vi "Format&SaveDataWithAttributes.vi"(0 "Comment":string="This is a test", 1 "Exp_Temperature_K":dbl=5.0, 2 "Det_Mono1_CenterWL_nm":dbl=490.0, 3 "Exc_ExcitationPower_uW":dbl=0.21, 4 "Exc_ExcitationSource":enum16{"P", "CW"}(ring), 5 "Exc_ExcitationWavelength_nm":dbl=450.0, 6 "Det_AcqTime_ms":dbl=500.0, 7 "Det_Mono1_EntSlit_mm":dbl=0.01, 8 "Measurement type":T2(ring)=enum."XY Intensity Map", 9 "Det_Mono1_ExtSlit_mm":dbl=0.01, 10 "Data_PLInt_cts":i32[](array[numeric])=[1, 3, 2, 1], 11 "FileName":string="test", 12 "Data_Wavelength_nm":sgl[](array[numeric])=[490.08, 490.12, 490.16, 490.2], 13 "Acq Mode":T1=enum."Spectrum" caption="Acq mode", 14 "Data_Angle_deg":sgl[](array[numeric])=[490.08, 490.12, 490.16, 490.2], 15 "Log File In":string, 16 "Data_FSMPos_V":dbl[][](array[numeric]), 18 "Data_CCD_px":dbl[][](array[numeric])) -> (17 "Log File Out":string, 25 "WrittenDatasetName":string)   [LabVIEW 2019]
uses:
  TypeDefs/AcqMode.ctl
  <vilib>/UPVI/lvhdf5/dataset.llb/LVH5D Operation.ctl
  <vilib>/Utility/miscctls.llb/LVRectTypeDef.ctl
  <vilib>/UPVI/lvhdf5/attribute.llb/LVH5A Operation.ctl
  <vilib>/UPVI/lvhdf5/group.llb/H5G_obj_t.ctl
  <vilib>/UPVI/lvhdf5/identifier.llb/Not an HDF5 Refnum Constant.vi
  <vilib>/UPVI/lvhdf5/common.llb/To HDF5 Ref.vi
  <vilib>/UPVI/lvhdf5/group.llb/OpenCreateGroup (String).vi
  <vilib>/Utility/VariantDataType/GetClusterInfo.vi
  <vilib>/Utility/VariantDataType/GetTypeInfo.vi
  <vilib>/UPVI/lvhdf5/utility.llb/Select HDF5 Dialog.vi
  <vilib>/UPVI/lvhdf5/utility.llb/Select HDF5 Dialog (Object Only).vi
  <vilib>/UPVI/lvhdf5/dataset.llb/Simple H5Dwrite (Variant).vi
  <vilib>/UPVI/lvhdf5/attribute.llb/Write Multiple Attributes.vi
  <vilib>/UPVI/lvhdf5/dataset.llb/H5Dclose.vi
  <vilib>/UPVI/lvhdf5/dataset.llb/Write Dataset with Attributes.xnode
  <vilib>/UPVI/lvhdf5/library.llb/HDF5 Ref.ctl
  <vilib>/UPVI/lvhdf5/attribute.llb/Cluster to Attribute Array.xnode
  <vilib>/Utility/error.llb/Error Cluster From Error Code.vi
  <vilib>/UPVI/lvhdf5/dataset.llb/OpenCreateReplace Dataset by Element Type.vi
  <vilib>/UPVI/lvhdf5/dataspace.llb/H5Sselect_hyperslab.vi
  <vilib>/UPVI/lvhdf5/dataset.llb/H5Dwrite (Variant).vi
  <vilib>/UPVI/lvhdf5/dataset.llb/H5Dget_space.vi
  <vilib>/UPVI/lvhdf5/attribute.llb/private/LVH5AwriteWDTAttrs.vi
  <vilib>/UPVI/lvhdf5/dataspace.llb/H5Sclose.vi
  <vilib>/UPVI/lvhdf5/file.llb/LVH5F Operation.ctl
  <vilib>/UPVI/lvhdf5/utility.llb/Select HDF5 Dialog (File and Object).vi
  <vilib>/Utility/VariantDataType/VariantType.lvlib
panel:
  in  "Main 3D Data to write":dbl[][][](array[numeric])=[[[2.2, 4.4, 3.3, 5.5, 6.6]]]
  out "File path":path=path "Cluster Attributes.hdf5"
  in  "DatasetName":string="test"
  in  "Main 2D Data to write":dbl[][](array[numeric])=[[2.2, 4.4, 3.3, 5.5, 6.6]]
  out "Date":string="2006-1-11"
  in  "Pol_L/2Exc_deg":dbl[](array[numeric])
  in  "Pol_L/2Det_deg":dbl[](array[numeric])
  in  "MeasurementName":string
  out "Exists":bool
  out "Homonyms":string[](array[string])
  out "size(s)":i32
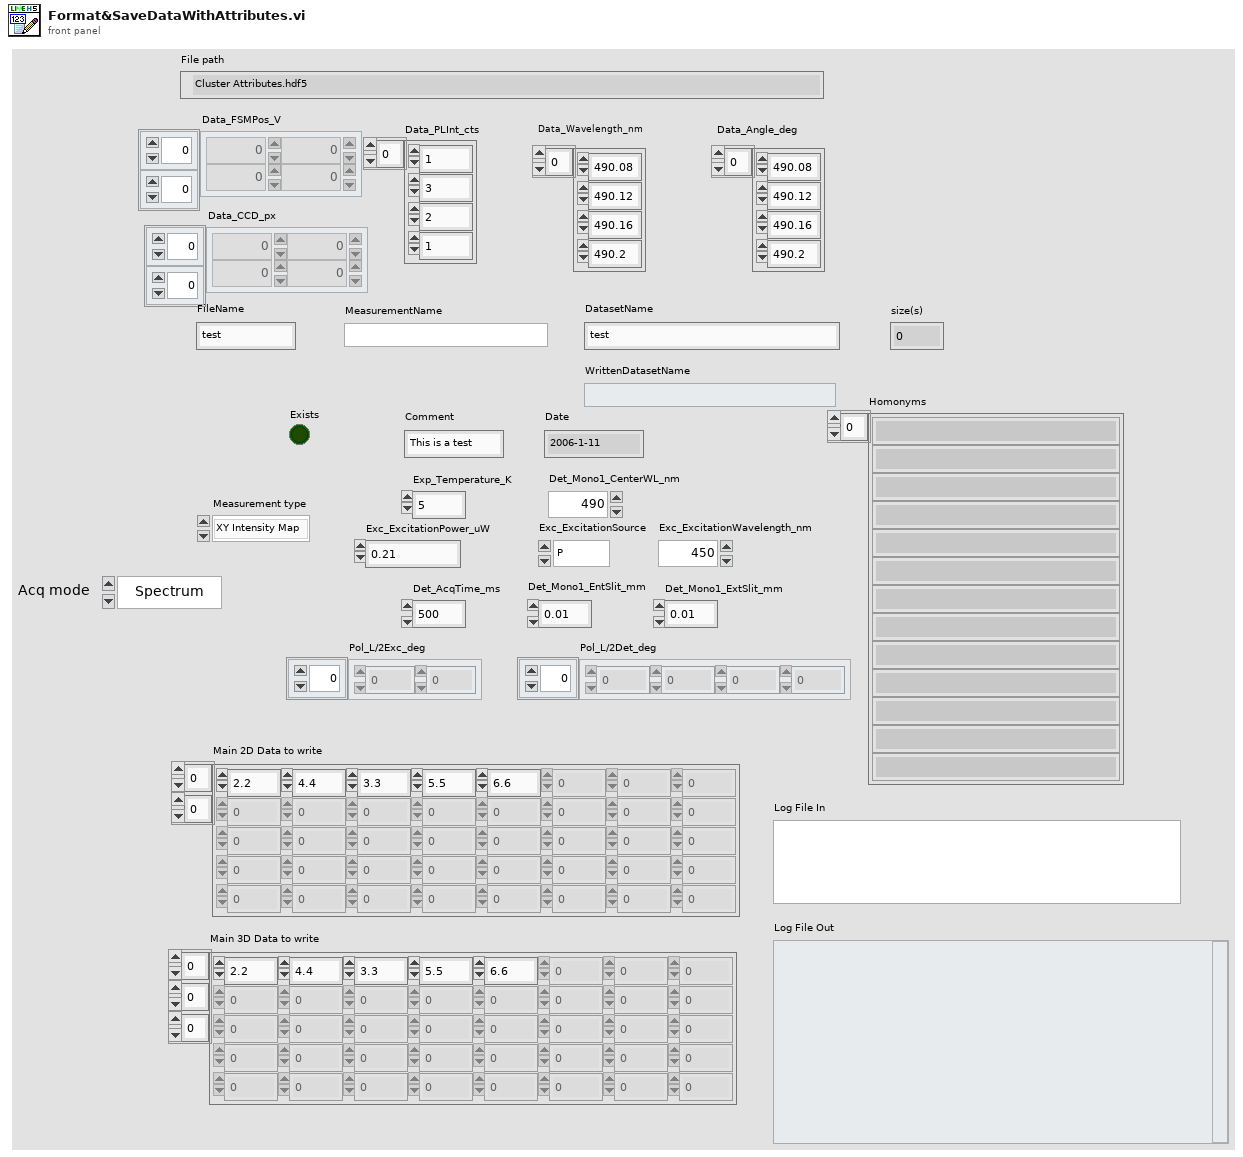
[diagram p1: front panel]
types:
  T1 = typedef "AcqMode.ctl" = enum16{"Image", "Spectrum", "APD 1", "APD 2", "APD 1+2"}
  T2 = enum16{"Contrast", "XY Intensity Map", "Polarisation", "Spectrum"}
  T3 = typedef "LVH5D Operation.ctl" = enum16{"open", "replace", "create", "open or create", "create or replace", "create or replace with confirmation"}
  T4 = typedef "HDF5 Ref.ctl" = refnum<k1>
  T5 = typedef "LVH5A Operation.ctl" = enum16{"open", "replace", "create", "open or create", "create or replace", "create or replace with confirmation"}
  T6 = typedef "LVRectTypeDef.ctl" = cluster{"Left":i16, "Top":i16, "Right":i16, "Bottom":i16}
  T7 = cluster{"Behavior":enum32{"Invalid", "Default", "Floating", "Floating/Auto-Hide", "Modal"}, "Position":T6, "Center":bool, "Title":string}
  T8 = typedef "LVH5F Operation.ctl" = enum16{"open", "open or create", "create or replace", "create or replace (with confirmation)", "create", "open (read only)"}
  T9 = typedef "H5G_obj_t.ctl" = i32
  T10 = cluster{"Object Types (any)":T9[], "Object Pattern":string}
  T11 = cluster{"date/time string":string, "Comment":string, "Exp_Temperature_K":dbl, "Exc_ExcitationSource":enum16{"P", "CW"}, "Exc_ExcitationWavelength_nm":dbl, "Exc_ExcitationPower_uW":dbl, "Det_AcqTime_ms":dbl, "Det_Mono1_EntSlit_mm":dbl, "Det_Mono1_ExtSlit_mm":dbl, "Pol_L/2Exc_deg":dbl[], "Pol_L/2Det_deg":dbl[], "Data_CCD_px":dbl[][]}
  T12 = cluster{"date/time string":string, "Comment":string, "Exp_Temperature_K":dbl, "Exc_ExcitationSource":enum16{"P", "CW"}, "Exc_ExcitationWavelength_nm":dbl, "Exc_ExcitationPower_uW":dbl, "Det_AcqTime_ms":dbl, "Det_Mono1_EntSlit_mm":dbl, "Det_Mono1_ExtSlit_mm":dbl, "Pol_L/2Exc_deg":dbl[], "Pol_L/2Det_deg":dbl[], "Data_Wavelength_nm":sgl[]}
  T13 = cluster{"date/time string":string, "Comment":string, "Exp_Temperature_K":dbl, "Exc_ExcitationSource":enum16{"P", "CW"}, "Exc_ExcitationWavelength_nm":dbl, "Exc_ExcitationPower_uW":dbl, "Det_AcqTime_ms":dbl, "Det_Mono1_EntSlit_mm":dbl, "Det_Mono1_ExtSlit_mm":dbl, "Pol_L/2Exc_deg":dbl[], "Pol_L/2Det_deg":dbl[], "Data_FSMPos_V":dbl[][]}
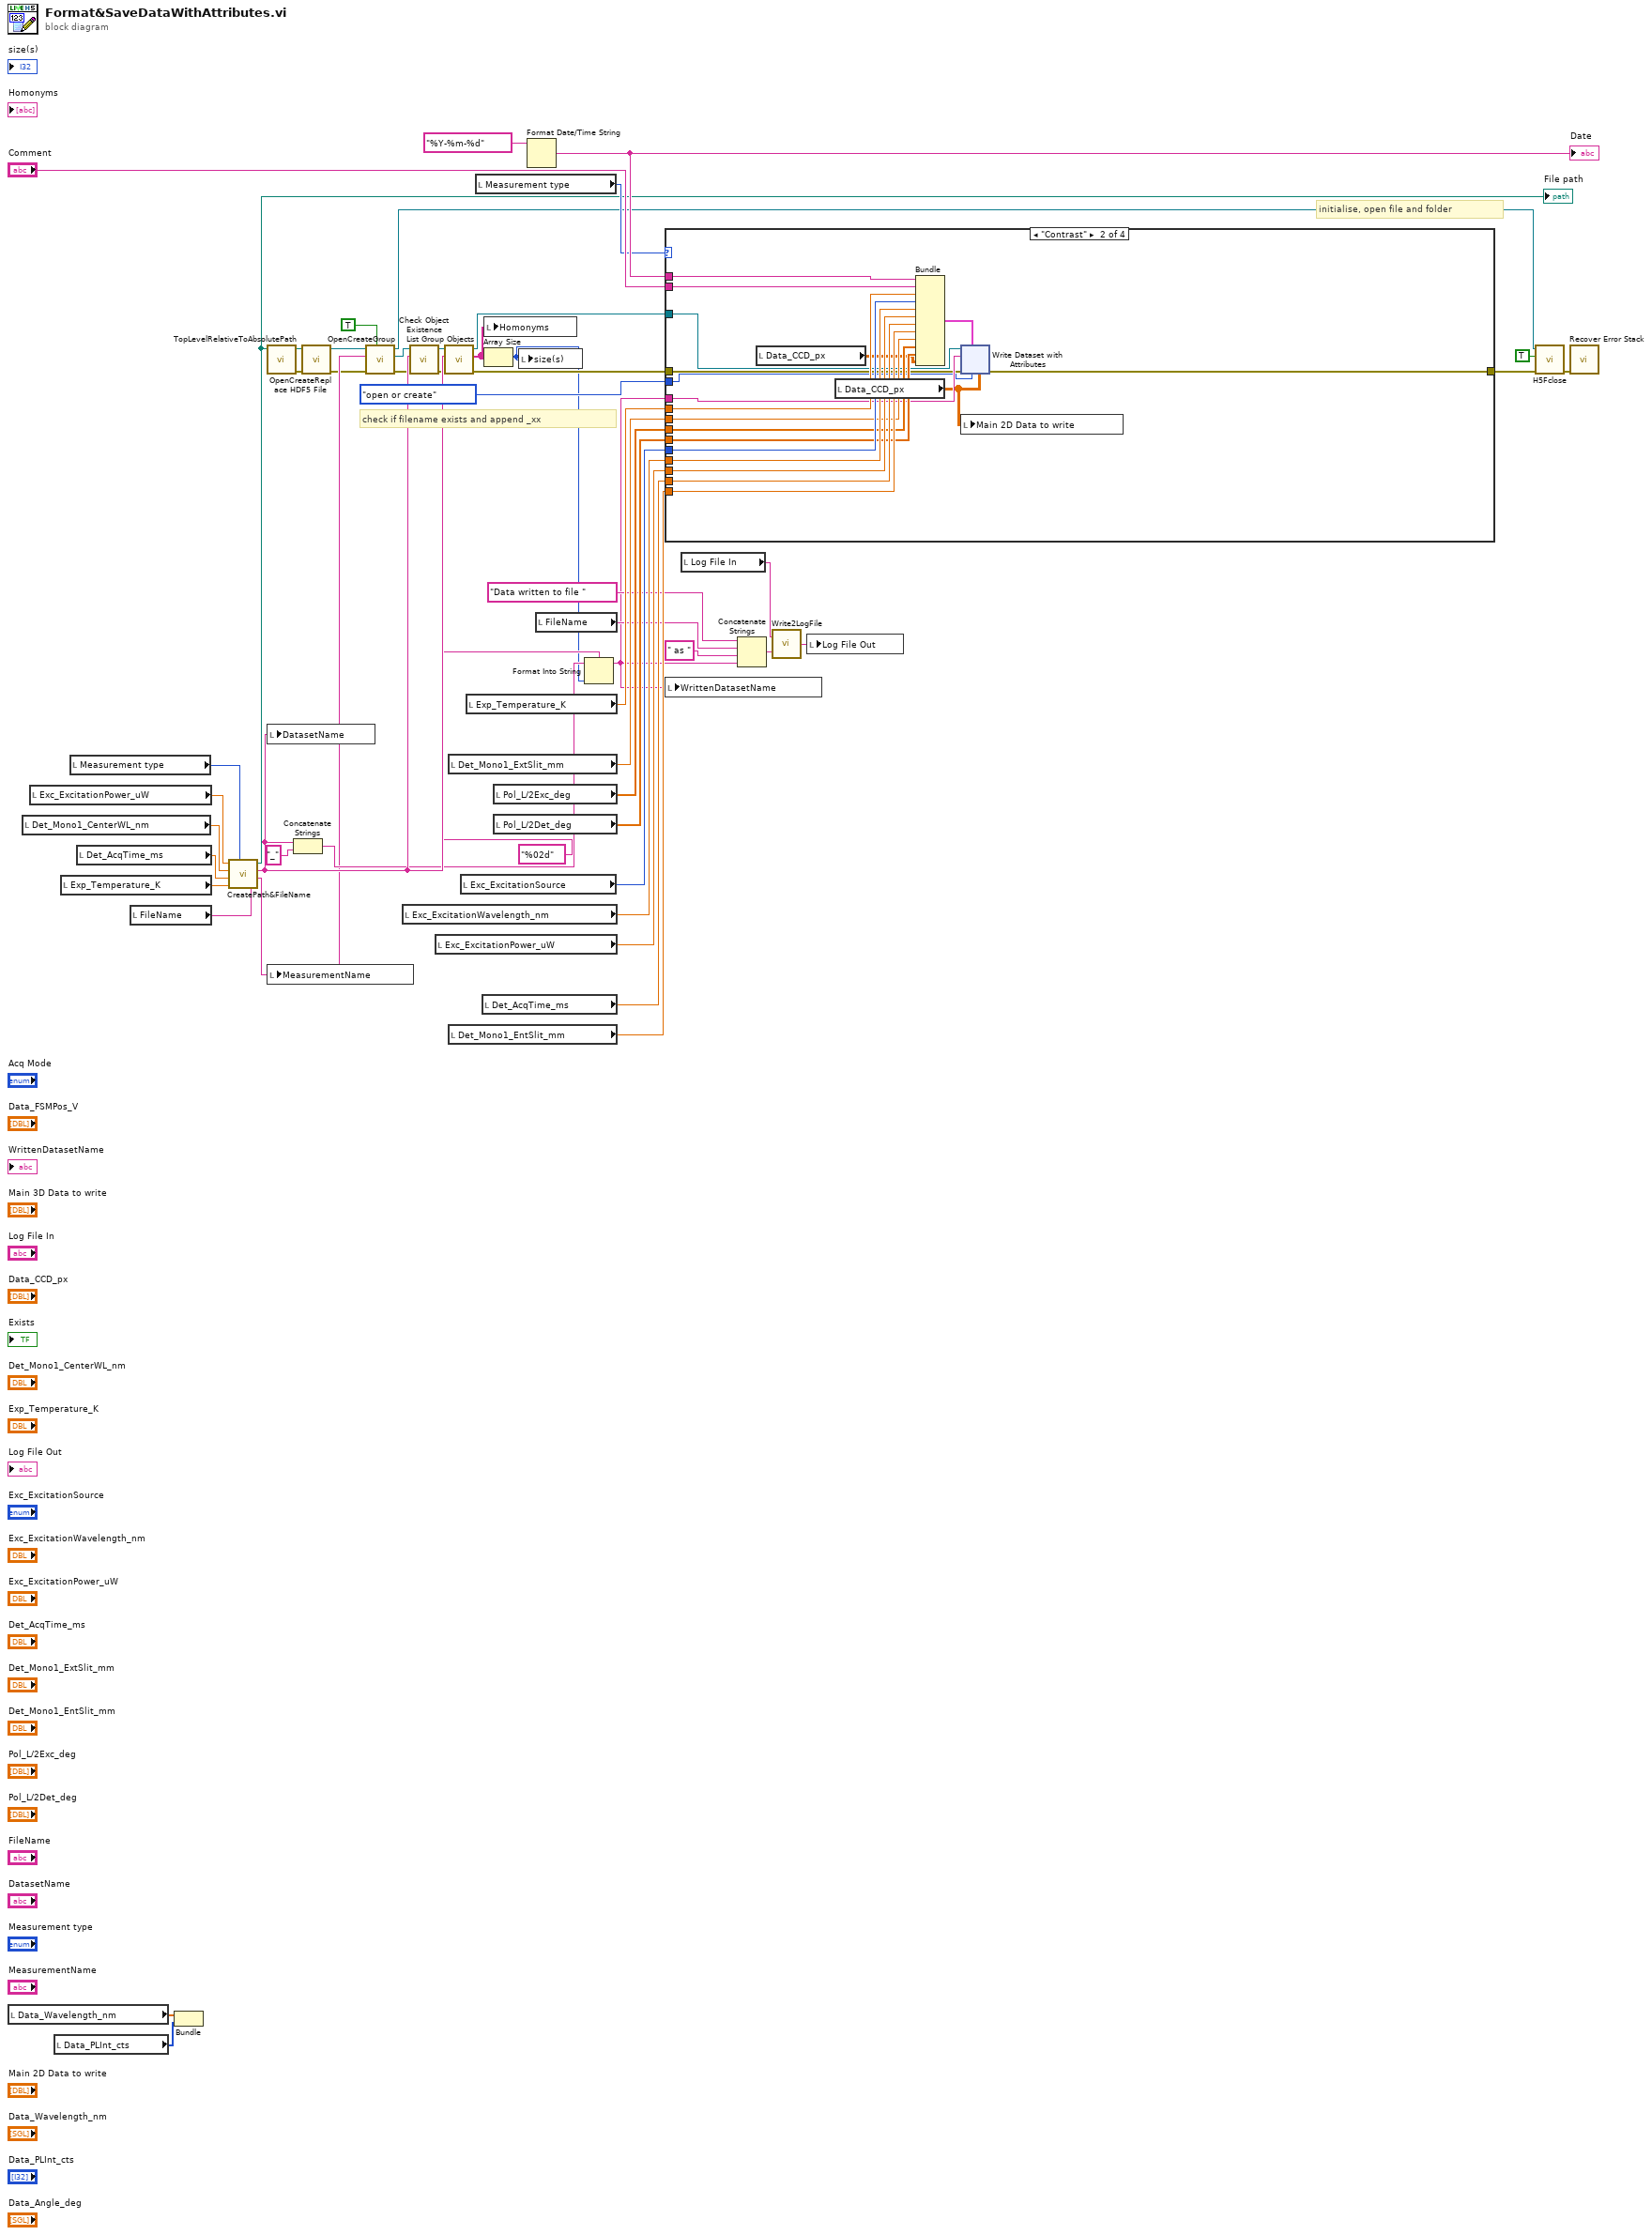
[diagram p0: block diagram]
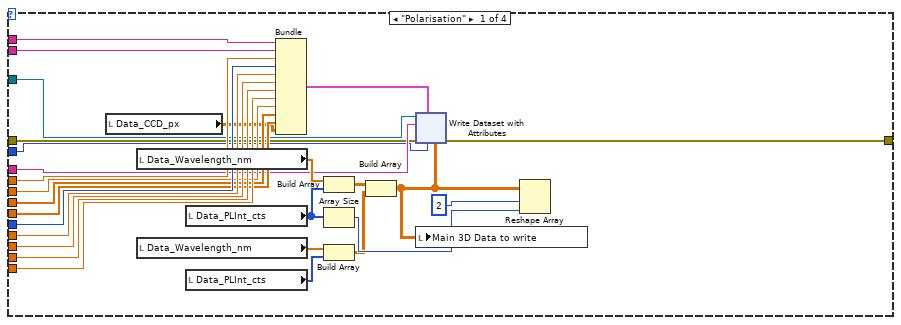
[diagram p2: hidden frame]
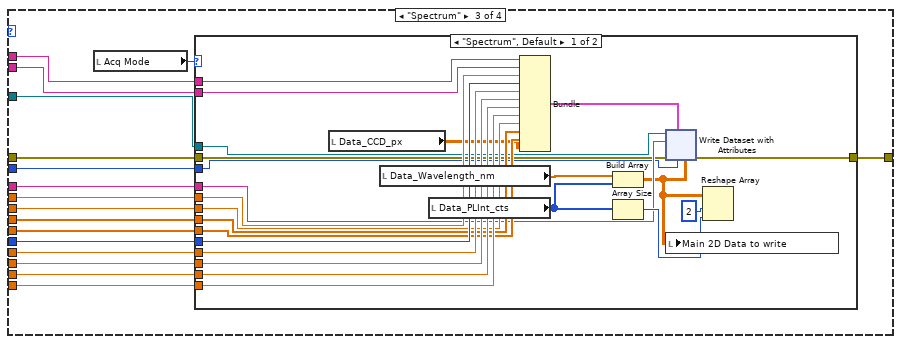
[diagram p3: hidden frame]
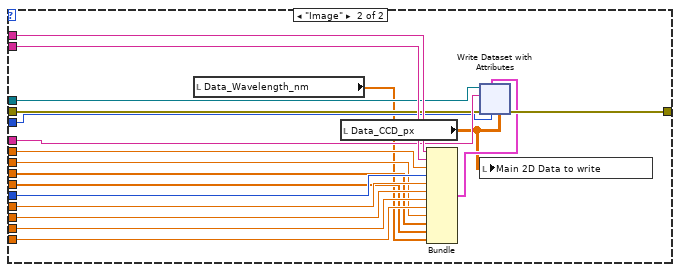
[diagram p4: hidden frame]
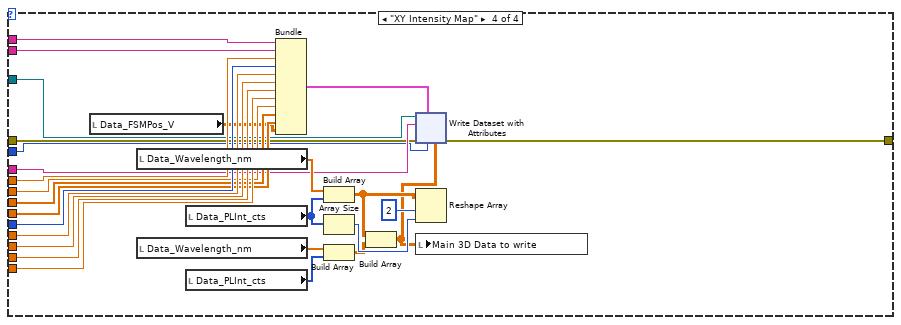
[diagram p5: hidden frame]
diagram:
  # "initialise, open file and folder"
  # "check if filename exists and append _xx"
  n1 = local read "Data_Wavelength_nm"() -> (w12:sgl[])
  n2 = local read "Det_Mono1_CenterWL_nm"() -> (w26:dbl)
  n3 = local read "Exc_ExcitationPower_uW"() -> (w23:dbl)
  n4 = local read "Data_PLInt_cts"() -> (w13:i32[])
  n5 = local read "Exp_Temperature_K"() -> (w24:dbl)
  n6 = local read "Measurement type"() -> (w1:T2)
  n7 = local read "Det_AcqTime_ms"() -> (w22:dbl)
  n8 = local read "FileName"() -> (w21:string)
  n9 = Bundle("Data_Wavelength_nm"=w12, "Data_PLInt_cts"=w13) -> ()  [unwired: 1 in, 1 out]
  n10 = call "CreatePath&FileName.vi"("FileName"=w21, "Measurement type"=w1, "Temp_K"=w24, "AcqTime_ms"=w22, "CenterWL_nm"=w26, "ExcPow_uW"=w23) -> ("MeasurementGroupName"=w25:string, "DatasetName"=w37:string, "File path"=w14:path)
  "File path" <- w14
  n11 = call "TopLevelRelativeToAbsolutePath.vi"("Path Relative to Top Level VI"=w14) -> ("error out"=w10:errorcluster, "Absolute path"=w9:path)  [unwired: 9 in]
  n12 = local write "DatasetName"(w37) -> ()
  n13 = local write "MeasurementName"(w25) -> ()
  n14 = Concatenate Strings(w37, "_" ("string")) -> (w35:string)
  n15 = call <vilib>:"OpenCreateReplace HDF5 File.vi"("error in (no error)"=w10, "path"=w9) -> ("error out"=w16:errorcluster, "HDF5 Ref out"=w15:T4)  [unwired: 6 in]
  n16 = call-poly <vilib>:"OpenCreateGroup.vi"("Create if not found (F)"=TRUE, "error in (no error)"=w16, "Group"=w25, "HDF5 Ref"=w15) -> ("error out"=w29:errorcluster, "HDF5 Group Ref"=w28:T4, "HDF5 Ref out"=w19:T4)  [unwired: 5 in]
  n17 = local read "Exc_ExcitationWavelength_nm"() -> (w42:dbl)
  n18 = call <vilib>:"Check Object Existence.vi"("error in (no error)"=w29, "name"=w37, "HDF5 Ref"=w28) -> ("error out"=w30:errorcluster, "HDF5 Ref out"=w31:T4)  [unwired: 4 in, 1 out]
  n19 = local read "Exc_ExcitationPower_uW"() -> (w43:dbl)
  n20 = call <vilib>:"List Group Objects.vi"("error in (no error)"=w30, "pattern"=w37, "HDF5 Loc Ref"=w31) -> ("error out"=w49:errorcluster, "Object Names"=w32:string[], "HDF5 Loc Ref out"=w51:T4)  [unwired: 3 in, 1 out]
  n21 = local read "Det_Mono1_ExtSlit_mm"() -> (w46:dbl)
  n22 = local read "Det_Mono1_EntSlit_mm"() -> (w45:dbl)
  n23 = local read "Exc_ExcitationSource"() -> (w41:enum16{"P", "CW"})
  n24 = local read "Exp_Temperature_K"() -> (w40:dbl)
  n25 = local read "Measurement type"() -> (w20:T2)
  n26 = local read "Det_AcqTime_ms"() -> (w44:dbl)
  n27 = local write "Homonyms"(w32) -> ()
  n28 = Array Size(array=w32) -> (size(s)=w34:i32)
  n29 = local read "Pol_L/2Exc_deg"() -> (w47:dbl[])
  n30 = local read "Pol_L/2Det_deg"() -> (w48:dbl[])
  n31 = local write "size(s)"(w34) -> ()
  n32 = Format Date/Time String(time format string (%c)="%Y-%m-%d") -> (date/time string=w38:string)  [unwired: 2 in]
  "Date" <- w38
  n33 = local read "FileName"() -> (w7:string)
  n34 = Format Into String(format string="%02d", initial string=w35, w34) -> (resulting string=w5:string)  [unwired: 1 in, 1 out]
  n35 = case shown="\"Contrast\"" w20 {
    tunnel: w38 -> [w75 w414 w747 w1444]
    tunnel: "Comment" -> [w74 w413 w746 w1443]
    tunnel: w40 -> [w73 w412 w745 w1442]
    tunnel: w41 -> [w72 w411 w744 w1441]
    tunnel: w42 -> [w71 w410 w743 w1440]
    tunnel: w43 -> [w70 w409 w742 w1439]
    tunnel: w44 -> [w69 w408 w741 w1438]
    tunnel: w45 -> [w68 w407 w740 w1437]
    tunnel: w46 -> [w67 w406 w739 w1436]
    tunnel: w47 -> [w66 w405 w738 w1435]
    tunnel: w48 -> [w65 w404 w737 w1434]
    tunnel: w5 -> [w64 w403 w736 w1433]
    tunnel: w49 -> [w63 w402 w735 w1432]
    tunnel: LVH5D_Operation."open or create" ("operation (open or create)") -> [w62 w401 w734 w1431]
    tunnel: w51 -> [w61 w400 w733 w1430]
    tunnel: [w60 w399 w732 w1429] -> w52
    frame "Polarisation" {
      n36 = local read "Data_CCD_px"() -> (w59:dbl[][])
      n37 = local read "Data_Wavelength_nm"() -> (w76:sgl[])
      n38 = local read "Data_Wavelength_nm"() -> (w57:sgl[])
      n39 = local read "Data_PLInt_cts"() -> (w77:i32[])
      n40 = local read "Data_PLInt_cts"() -> (w56:i32[])
      n41 = Bundle("date/time string"=w75, "Comment"=w74, "Exp_Temperature_K"=w73, "Exc_ExcitationSource"=w72, "Exc_ExcitationWavelength_nm"=w71, "Exc_ExcitationPower_uW"=w70, "Det_AcqTime_ms"=w69, "Det_Mono1_EntSlit_mm"=w68, "Det_Mono1_ExtSlit_mm"=w67, "Pol_L/2Exc_deg"=w66, "Pol_L/2Det_deg"=w65, "Data_CCD_px"=w59) -> (w58:T11)  [unwired: 1 in]
      n42 = Build Array(w76, w77) -> (w54:sgl[][])
      n43 = Array Size(array=w77) -> (size(s)=w78:i32)
      n44 = Build Array(w57, w56) -> (w55:sgl[][])
      n45 = Build Array(w54, w55) -> (w53:sgl[][][])
      n46 = xnode "Write Dataset with Attributes"("Dataset Path"=w64, "error in (no error)"=w63, "operation (open or create)"=w62, "HDF5 Path or Ref"=w61, "Attribute Value(s)"=w58, "Data"=w53) -> ("error out"=w60:errorcluster)  [unwired: 2 in, 2 out]
      n47 = local write "Main 3D Data to write"(w53) -> ()
      n48 = Reshape Array(w53, 2 ("dimension size"), w78) -> ()  [unwired: 1 out]
    }
    frame "Contrast" {
      n49 = local read "Data_CCD_px"() -> (w398:dbl[][])
      n50 = local read "Data_CCD_px"() -> (w396:dbl[][])
      n51 = Bundle("date/time string"=w414, "Comment"=w413, "Exp_Temperature_K"=w412, "Exc_ExcitationSource"=w411, "Exc_ExcitationWavelength_nm"=w410, "Exc_ExcitationPower_uW"=w409, "Det_AcqTime_ms"=w408, "Det_Mono1_EntSlit_mm"=w407, "Det_Mono1_ExtSlit_mm"=w406, "Pol_L/2Exc_deg"=w405, "Pol_L/2Det_deg"=w404, "Data_CCD_px"=w398) -> (w397:T11)  [unwired: 1 in]
      n52 = xnode "Write Dataset with Attributes"("Dataset Path"=w403, "error in (no error)"=w402, "operation (open or create)"=w401, "HDF5 Path or Ref"=w400, "Attribute Value(s)"=w397, "Data"=w396) -> ("error out"=w399:errorcluster)  [unwired: 2 in, 2 out]
      n53 = local write "Main 2D Data to write"(w396) -> ()
    }
    frame "Spectrum" {
      n54 = local read "Acq Mode"() -> (w731:T1)
      n55 = case shown="\"Spectrum\", Default" w731 {
        tunnel: w747 -> [w766 w1105]
        tunnel: w746 -> [w765 w1104]
        tunnel: w745 -> [w764 w1103]
        tunnel: w744 -> [w763 w1102]
        tunnel: w743 -> [w762 w1101]
        tunnel: w742 -> [w761 w1100]
        tunnel: w741 -> [w760 w1099]
        tunnel: w740 -> [w759 w1098]
        tunnel: w739 -> [w758 w1097]
        tunnel: w738 -> [w757 w1096]
        tunnel: w737 -> [w756 w1095]
        tunnel: w736 -> [w755 w1094]
        tunnel: w735 -> [w754 w1093]
        tunnel: w734 -> [w753 w1092]
        tunnel: w733 -> [w752 w1091]
        tunnel: [w751 w1090] -> w732
        frame "Spectrum", Default {
          n56 = local read "Data_CCD_px"() -> (w750:dbl[][])
          n57 = local read "Data_Wavelength_nm"() -> (w767:sgl[])
          n58 = local read "Data_PLInt_cts"() -> (w768:i32[])
          n59 = Bundle("date/time string"=w766, "Comment"=w765, "Exp_Temperature_K"=w764, "Exc_ExcitationSource"=w763, "Exc_ExcitationWavelength_nm"=w762, "Exc_ExcitationPower_uW"=w761, "Det_AcqTime_ms"=w760, "Det_Mono1_EntSlit_mm"=w759, "Det_Mono1_ExtSlit_mm"=w758, "Pol_L/2Exc_deg"=w757, "Pol_L/2Det_deg"=w756, "Data_CCD_px"=w750) -> (w749:T11)  [unwired: 1 in]
          n60 = Build Array(w767, w768) -> (w748:sgl[][])
          n61 = Array Size(array=w768) -> (size(s)=w769:i32)
          n62 = xnode "Write Dataset with Attributes"("Dataset Path"=w755, "error in (no error)"=w754, "operation (open or create)"=w753, "HDF5 Path or Ref"=w752, "Attribute Value(s)"=w749, "Data"=w748) -> ("error out"=w751:errorcluster)  [unwired: 2 in, 2 out]
          n63 = local write "Main 2D Data to write"(w748) -> ()
          n64 = Reshape Array(w748, 2 ("dimension size"), w769) -> ()  [unwired: 1 out]
        }
        frame "Image" {
          n65 = local read "Data_Wavelength_nm"() -> (w1089:sgl[])
          n66 = local read "Data_CCD_px"() -> (w1087:dbl[][])
          n67 = Bundle("date/time string"=w1105, "Comment"=w1104, "Exp_Temperature_K"=w1103, "Exc_ExcitationSource"=w1102, "Exc_ExcitationWavelength_nm"=w1101, "Exc_ExcitationPower_uW"=w1100, "Det_AcqTime_ms"=w1099, "Det_Mono1_EntSlit_mm"=w1098, "Det_Mono1_ExtSlit_mm"=w1097, "Pol_L/2Exc_deg"=w1096, "Pol_L/2Det_deg"=w1095, "Data_Wavelength_nm"=w1089) -> (w1088:T12)  [unwired: 1 in]
          n68 = xnode "Write Dataset with Attributes"("Dataset Path"=w1094, "error in (no error)"=w1093, "operation (open or create)"=w1092, "HDF5 Path or Ref"=w1091, "Attribute Value(s)"=w1088, "Data"=w1087) -> ("error out"=w1090:errorcluster)  [unwired: 2 in, 2 out]
          n69 = local write "Main 2D Data to write"(w1087) -> ()
        }
      }
    }
    frame "XY Intensity Map" {
      n70 = local read "Data_FSMPos_V"() -> (w1428:dbl[][])
      n71 = local read "Data_Wavelength_nm"() -> (w1445:sgl[])
      n72 = local read "Data_Wavelength_nm"() -> (w1426:sgl[])
      n73 = local read "Data_PLInt_cts"() -> (w1446:i32[])
      n74 = local read "Data_PLInt_cts"() -> (w1422:i32[])
      n75 = Bundle("date/time string"=w1444, "Comment"=w1443, "Exp_Temperature_K"=w1442, "Exc_ExcitationSource"=w1441, "Exc_ExcitationWavelength_nm"=w1440, "Exc_ExcitationPower_uW"=w1439, "Det_AcqTime_ms"=w1438, "Det_Mono1_EntSlit_mm"=w1437, "Det_Mono1_ExtSlit_mm"=w1436, "Pol_L/2Exc_deg"=w1435, "Pol_L/2Det_deg"=w1434, "Data_FSMPos_V"=w1428) -> (w1427:T13)  [unwired: 1 in]
      n76 = Build Array(w1445, w1446) -> (w1424:sgl[][])
      n77 = Array Size(array=w1446) -> (size(s)=w1447:i32)
      n78 = Build Array(w1426, w1422) -> (w1425:sgl[][])
      n79 = Build Array(w1424, w1425) -> (w1423:sgl[][][])
      n80 = xnode "Write Dataset with Attributes"("Dataset Path"=w1433, "error in (no error)"=w1432, "operation (open or create)"=w1431, "HDF5 Path or Ref"=w1430, "Attribute Value(s)"=w1427, "Data"=w1423) -> ("error out"=w1429:errorcluster)  [unwired: 2 in, 2 out]
      n81 = Reshape Array(w1424, 2 ("dimension size"), w1447) -> ()  [unwired: 1 out]
      n82 = local write "Main 3D Data to write"(w1423) -> ()
    }
  }
  n83 = local write "WrittenDatasetName"(w5) -> ()
  n84 = local read "Log File In"() -> (w4:string)
  n85 = Concatenate Strings("Data written to file ", w7, " as ", w5) -> (w3:string)
  n86 = call "Write2LogFile.vi"("Add to log file"=w3, "Log file before"=w4) -> ("Log file after"=w2:string)
  n87 = local write "Log File Out"(w2) -> ()
  n88 = call <vilib>:"H5Fclose.vi"("error in (no error)"=w52, "Close All Open Objects (T)"=TRUE, "HDF5 Ref"=w19) -> ("error out"=w17:errorcluster)  [unwired: 6 in]
  n89 = call <vilib>:"Recover Error Stack.vi"("error in (no error)"=w17) -> ()  [unwired: 5 in, 4 out]
